vi "PPAS_SIM_ENCODER_OPEN.vi"(4 "DistancePerCount":dbl, 8 "error in (no error)":errorcluster, 9 "Invert":bool, 10 "DIO Channel B":T1, 11 "DIO Channel  A":T1) -> (0 "error out":errorcluster, 3 "SwerveDriveEnc":T2)   [LabVIEW 2019]
uses:
  <vilib>/Rock Robotics/WPI/Encoder/WPI_EncoderDevRef.ctl
  <vilib>/Rock Robotics/SystemInterfaces/Encoder/FPGA_EncoderIdx.ctl
  <vilib>/Rock Robotics/SystemInterfaces/Counter/FPGA_CounterCtrSystemIndex.ctl
  <vilib>/Rock Robotics/WPI/Encoder/WPI_EncoderType.ctl
  <vilib>/Rock Robotics/SystemInterfaces/DIO/FPGA_DIOChannel.ctl
panel:
  in  "FPGA_Time_Seconds":dbl=-1.0
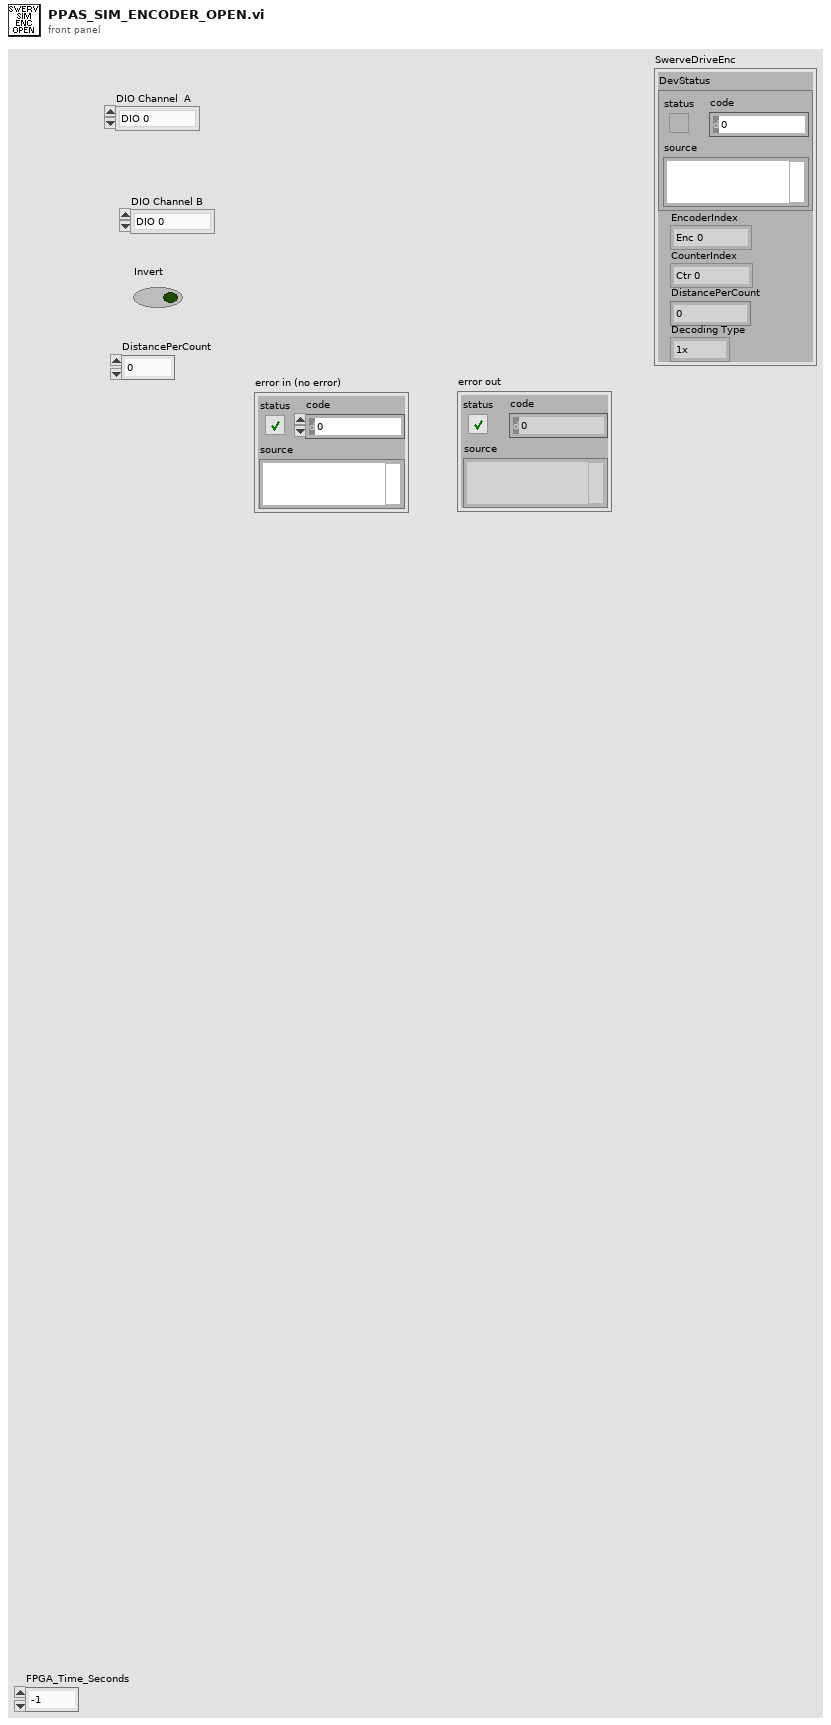
[diagram p1: front panel]
types:
  T1 = typedef "FPGA_DIOChannel.ctl" = enum8{"DIO 0", "DIO 1", "DIO 2", "DIO 3", "DIO 4", "DIO 5", "DIO 6", "DIO 7", "DIO 8", "DIO 9", "DIO MXP 0", "DIO MXP 1", "DIO MXP 2", "DIO MXP 3", "DIO MXP 4", "DIO MXP 5", "DIO MXP 6", "DIO MXP 7", "DIO MXP 8", "DIO MXP 9", "DIO MXP 10", "DIO MXP 11", "DIO MXP 12", "DIO MXP 13", "DIO MXP 14", "DIO MXP 15", "SPI Port CS1", "SPI Port CS2", "SPI Port CS3", "SPI Port MISO", "SPI Port MOSI", "Invalid"}
  T2 = typedef "WPI_EncoderDevRef.ctl" = cluster{"DevStatus":errorcluster, "EncoderIndex":T3, "CounterIndex":T4, "DistancePerCount":dbl, "Decoding Type":T5}
  T3 = typedef "FPGA_EncoderIdx.ctl" = enum8{"Enc 0", "Enc 1", "Enc 2", "Enc 3", "Enc 4", "Enc 5", "Enc 6", "Enc 7", "Invalid"}
  T4 = typedef "FPGA_CounterCtrSystemIndex.ctl" = enum8{"Ctr 0", "Ctr 1", "Ctr 2", "Ctr 3", "Ctr 4", "Ctr 5", "Ctr 6", "Ctr 7", "Invalid"}
  T5 = typedef "WPI_EncoderType.ctl" = enum16{"1x", "2x", "4x"}
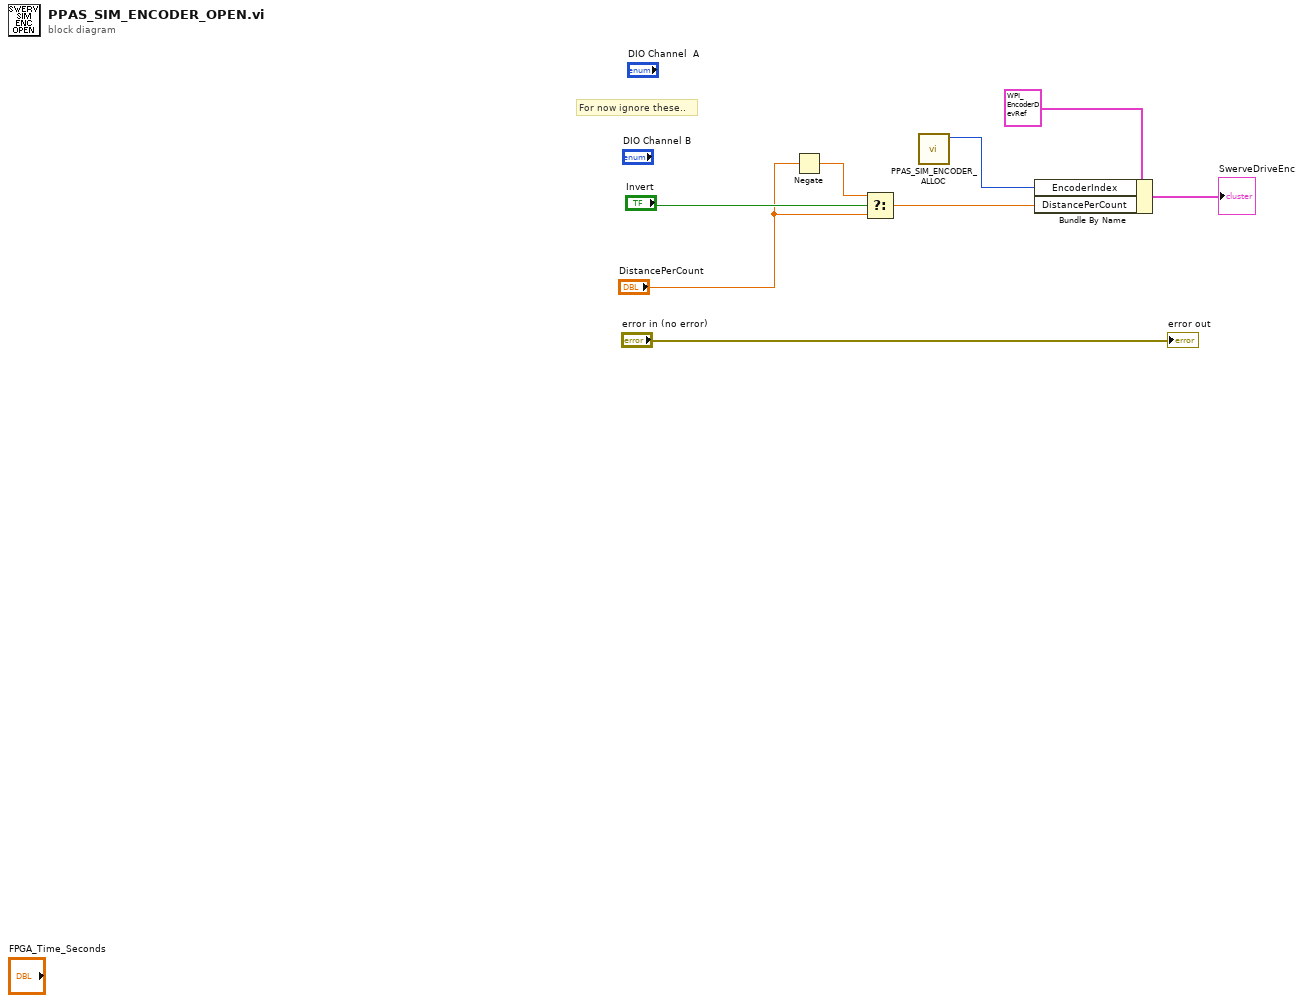
[diagram p0: block diagram]
diagram:
  # "For now ignore these.."
  n1 = Negate(x="DistancePerCount") -> (-x=w5:dbl)
  n2 = Select(t=w5, s="Invert", f="DistancePerCount") -> (s? t:f=w3:dbl)
  n3 = call "PPAS_SIM_ENCODER_ALLOC.vi"() -> ("Encoder Index"=w1:T3)  [unwired: 11 in]
  n4 = Bundle By Name(cluster=T2 {"DevStatus"={"status"=FALSE, "code"=0, "source"=""}, "EncoderIndex"=enum."Enc 0", "CounterIndex"=enum."Ctr 0", "DistancePerCount"=0.0, "Decoding Type"=enum."1x"} ("SwerveDriveEnc"), "EncoderIndex"=w1, "DistancePerCount"=w3) -> (→"SwerveDriveEnc":T2)
  "error out" <- "error in (no error)"
